vi "Test.vi"   [LabVIEW 2018]
doc: "This VI is called when test mode begins, and will automatically be terminated when it ends. You can add manual or automatic tests and invoke them from the dashboard."
uses:
  <vilib>/Rock Robotics/WPI/ThirdParty/Phoenix-LabVIEW/Motor Controller/Controls/CTRE_Phoenix_MotorControl_ControlMode.ctl
  <vilib>/Rock Robotics/WPI/Utilities/WPI_GetSetVariantRefNum.vi
  <vilib>/Rock Robotics/Network Tables/NT Read Number.vi
  <vilib>/Rock Robotics/WPI/RobotDrive/WPI_RobotDriveArcadeDrive_Standard(NoSaturation).vi
types:
  T1 = typedef "WPI_RobotDriveDevRef.ctl" = cluster{"DevStatus":errorcluster, "Motors[]":T2[], "Square Inputs":bool, "Max Output":dbl}
  T2 = typedef "WPI_MotorControlDeviceRef.ctl" = cluster{"DeviceStatus":errorcluster, "Type":T3, "PWM":cluster{"PWM Channel":T4, "DeadBand":T5}, "CAN":cluster{"Device Number":u8, "SetOutput VI Ref":variant, "GetOutput VI Ref":variant, "Enable VI Ref":variant, "Disable VI Ref":variant, "Data":variant}, "Invert":bool, "DIO PWM":cluster{"PWM \"Enable\" Channel":T4, "DIOChannel":T6, "PWM Rate":dbl}}
  T3 = typedef "WPI_MotorControlType.ctl" = enum16{"PWM", "CAN", "DIO PWM"}
  T4 = typedef "FPGA_DIOPWMChannel.ctl" = enum8{"PWM 0", "PWM 1", "PWM 2", "PWM 3", "PWM 4", "PWM 5", "PWM 6", "PWM 7", "PWM 8", "PWM 9", "PWM MXP 0", "PWM MXP 1", "PWM MXP 2", "PWM MXP 3", "PWM MXP 4", "PWM MXP 5", "PWM MXP 6", "PWM MXP 7", "PWM MXP 8", "PWM MXP 9", "Invalid"}
  T5 = typedef "WPI_PWMDeadband.ctl" = cluster{"Name":string, "maxPositivePwm":i32, "minPositivePwm":i32, "centerPwm":i32, "maxNegativePwm":i32, "minNegativePwm":i32, "angularRange":u16}
  T6 = typedef "FPGA_DIOChannel.ctl" = enum8{"DIO 0", "DIO 1", "DIO 2", "DIO 3", "DIO 4", "DIO 5", "DIO 6", "DIO 7", "DIO 8", "DIO 9", "DIO MXP 0", "DIO MXP 1", "DIO MXP 2", "DIO MXP 3", "DIO MXP 4", "DIO MXP 5", "DIO MXP 6", "DIO MXP 7", "DIO MXP 8", "DIO MXP 9", "DIO MXP 10", "DIO MXP 11", "DIO MXP 12", "DIO MXP 13", "DIO MXP 14", "DIO MXP 15", "SPI Port CS1", "SPI Port CS2", "SPI Port CS3", "SPI Port MISO", "SPI Port MOSI", "Invalid"}
  T7 = typedef "WPI_JoystickDevRef.ctl" = cluster{"Device":T8}
  T8 = typedef "WPI_JoystickDeviceEnum.ctl" = enum16{"USB 0", "USB 1", "USB 2", "USB 3", "USB 4", "USB 5"}
  T9 = cluster{"PhoenixMotorControlDevRef":T2, "PhoenixMotorControlDevRef":T2, "PhoenixMotorControlDevRef":T2, "MotorControlDevRef":T2, "MotorControlDevRef":T2, "RobotDriveDevRef":T1, "JoystickDevRef":T7}
  T10 = typedef "CTRE_Phoenix_MotorControl_ControlMode.ctl" = u16
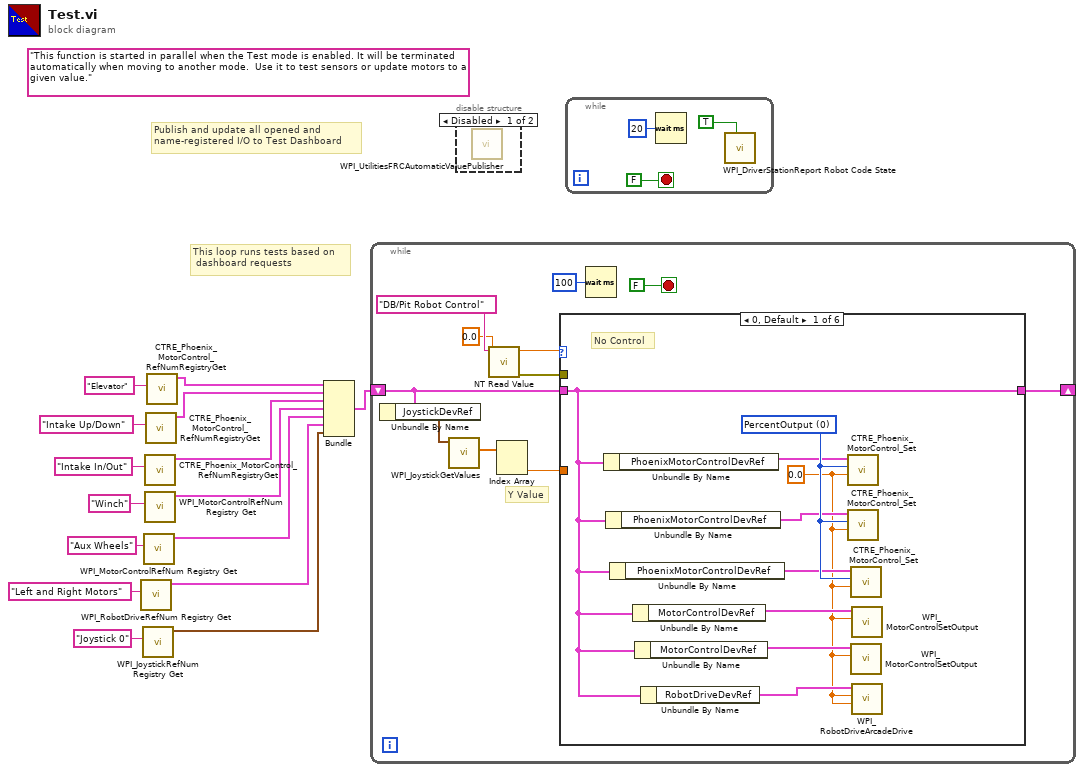
[diagram p0: block diagram]
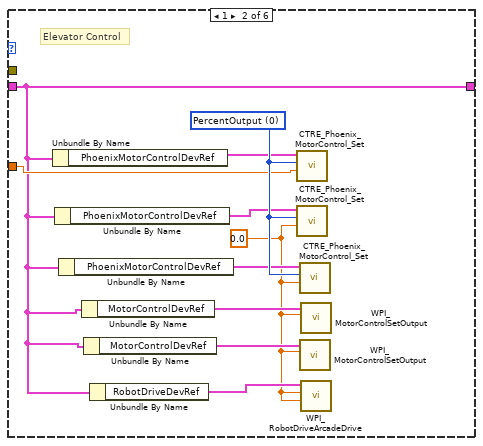
[diagram p2: hidden frame]
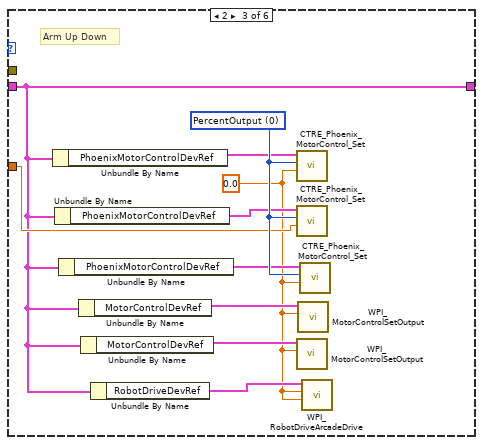
[diagram p3: hidden frame]
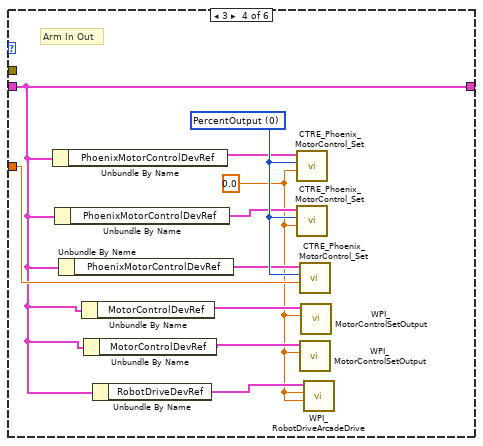
[diagram p4: hidden frame]
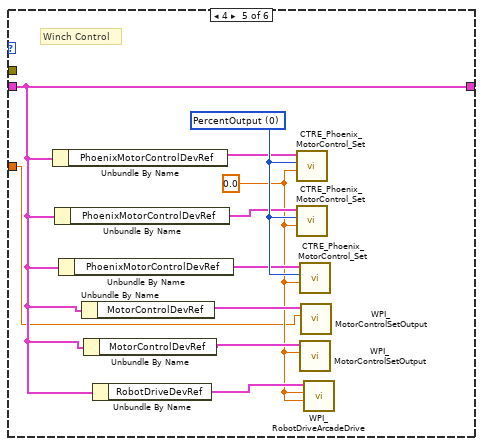
[diagram p5: hidden frame]
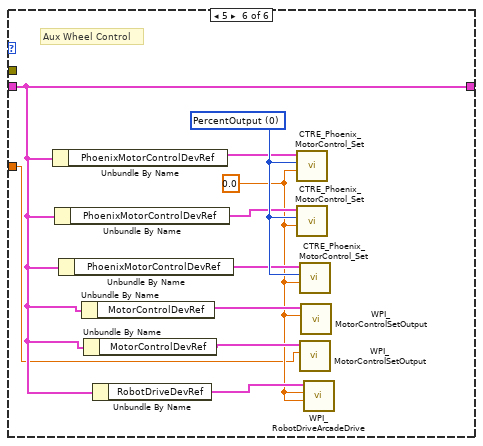
[diagram p6: hidden frame]
diagram:
  (unwired) "This function is started in parallel when the Test mode is enabled. It will be terminated automatically when moving to another mode.  Use it to test sensors or update motors to a given value."
  # "This loop runs tests based on \n dashboard requests"
  # "Publish and update all opened and\nname-registered I/O to Test Dashboard"
  n1 = call <vilib>:"WPI_RobotDriveRefNum Registry Get.vi"("refnum name"="Left and Right Motors") -> ("RobotDriveDevRef"=w6:T1)  [unwired: 9 in, 1 out]
  n2 = call <vilib>:"WPI_JoystickRefNum Registry Get.vi"("refnum name"="Joystick 0") -> ("JoystickDevRef"=w5:T7)  [unwired: 1 in, 9 out]
  n3 = call <vilib>:"WPI_MotorControlRefNum Registry Get.vi"("refnum name"="Aux Wheels") -> ("MotorControlDevRef"=w1:T2)  [unwired: 9 in, 1 out]
  n4 = call <vilib>:"CTRE_Phoenix_MotorControl_RefNumRegistryGet.vi"("refnum name"="Intake In/Out") -> ("PhoenixMotorControlDevRef"=w7:T2)  [unwired: 9 in, 1 out]
  n5 = call <vilib>:"WPI_MotorControlRefNum Registry Get.vi"("refnum name"="Winch") -> ("MotorControlDevRef"=w2:T2)  [unwired: 9 in, 1 out]
  n6 = call <vilib>:"CTRE_Phoenix_MotorControl_RefNumRegistryGet.vi"("refnum name"="Intake Up/Down") -> ("PhoenixMotorControlDevRef"=w8:T2)  [unwired: 9 in, 1 out]
  n7 = call <vilib>:"CTRE_Phoenix_MotorControl_RefNumRegistryGet.vi"("refnum name"="Elevator") -> ("PhoenixMotorControlDevRef"=w12:T2)  [unwired: 9 in, 1 out]
  n8 = Bundle("PhoenixMotorControlDevRef"=w12, "PhoenixMotorControlDevRef"=w8, "PhoenixMotorControlDevRef"=w7, "MotorControlDevRef"=w2, "MotorControlDevRef"=w1, "RobotDriveDevRef"=w6, "JoystickDevRef"=w5) -> (w13:T9)  [unwired: 1 in]
  n9 = while {
    shift-right: [w22] -> _
    shift-left: w13 -> [w19]
    stop <- FALSE stop-if-true
    # "Y Value"
    n10 = Unbundle By Name(w19) -> ("JoystickDevRef"=w18:T7)
    n11 = call <vilib>:"WPI_JoystickGetValues.vi"("JoystickDevRef"=w18) -> ("Axes"=w17:dbl[])  [unwired: 6 in, 4 out]
    n12 = call-poly <vilib>:"NT Read Value.vi"("Default Value"=0.0, "Name"="DB/Pit Robot Control") -> ("error out"=w23:errorcluster, "Numeric"=w24:dbl)  [unwired: 8 in]
    n13 = Index Array(array=w17) -> (element #2=w16:dbl)  [unwired: 2 in, 1 out]
    n14 = case shown="0, Default" w24 {
      tunnel: w23 -> [_ _ _ _ _ _]
      tunnel: w19 -> [w27 w39 w49 w59 w70 w80]
      tunnel: [w27 w39 w49 w59 w70 w80] -> w22
      tunnel: w16 -> [_ w40 w50 w60 w66 w76]
      frame 0, Default {
        w28 = 0.0 ("Output")
        w35 = T10 0 items=["PercentOutput"=0, "Position"=1, "Velocity"=2, "Current"=3, "Follower"=5, "MotionProfile"=6, "MotionMagic"=7, "MotionProfileArc"=10, "Disabled"=15] ("Control Mode")
        # "No Control"
        n15 = Unbundle By Name(w27) -> ("PhoenixMotorControlDevRef"=w34:T2)
        n16 = Unbundle By Name(w27) -> ("PhoenixMotorControlDevRef"=w31:T2)
        n17 = Unbundle By Name(w27) -> ("PhoenixMotorControlDevRef"=w32:T2)
        n18 = Unbundle By Name(w27) -> ("MotorControlDevRef"=w30:T2)
        n19 = Unbundle By Name(w27) -> ("MotorControlDevRef"=w29:T2)
        n20 = Unbundle By Name(w27) -> ("RobotDriveDevRef"=w33:T1)
        n21 = call <vilib>:"CTRE_Phoenix_MotorControl_Set.vi"("Output"=w28, "Control Mode"=w35, "PhoenixMotorControlDevRef"=w34) -> ()  [unwired: 7 in, 2 out]
        n22 = call <vilib>:"CTRE_Phoenix_MotorControl_Set.vi"("Output"=w28, "Control Mode"=w35, "PhoenixMotorControlDevRef"=w31) -> ()  [unwired: 7 in, 2 out]
        n23 = call <vilib>:"CTRE_Phoenix_MotorControl_Set.vi"("Output"=w28, "Control Mode"=w35, "PhoenixMotorControlDevRef"=w32) -> ()  [unwired: 7 in, 2 out]
        n24 = call <vilib>:"WPI_MotorControlSetOutput.vi"("Output"=w28, "MotorControlDevRef"=w29) -> ()  [unwired: 7 in, 3 out]
        n25 = call <vilib>:"WPI_MotorControlSetOutput.vi"("Output"=w28, "MotorControlDevRef"=w30) -> ()  [unwired: 7 in, 3 out]
        n26 = call-poly <vilib>:"WPI_RobotDriveArcadeDrive.vi"("Y axis value"=w28, "X axis value"=w28, "RobotDriveDevRef"=w33) -> ()  [unwired: 6 in, 3 out]
      }
      frame 1 {
        w36 = 0.0 ("Output")
        w45 = T10 0 items=["PercentOutput"=0, "Position"=1, "Velocity"=2, "Current"=3, "Follower"=5, "MotionProfile"=6, "MotionMagic"=7, "MotionProfileArc"=10, "Disabled"=15] ("Control Mode")
        # "Elevator Control"
        n27 = Unbundle By Name(w39) -> ("PhoenixMotorControlDevRef"=w44:T2)
        n28 = Unbundle By Name(w39) -> ("PhoenixMotorControlDevRef"=w41:T2)
        n29 = Unbundle By Name(w39) -> ("PhoenixMotorControlDevRef"=w42:T2)
        n30 = Unbundle By Name(w39) -> ("MotorControlDevRef"=w38:T2)
        n31 = Unbundle By Name(w39) -> ("MotorControlDevRef"=w37:T2)
        n32 = Unbundle By Name(w39) -> ("RobotDriveDevRef"=w43:T1)
        n33 = call <vilib>:"CTRE_Phoenix_MotorControl_Set.vi"("Output"=w40, "Control Mode"=w45, "PhoenixMotorControlDevRef"=w44) -> ()  [unwired: 7 in, 2 out]
        n34 = call <vilib>:"CTRE_Phoenix_MotorControl_Set.vi"("Output"=w36, "Control Mode"=w45, "PhoenixMotorControlDevRef"=w41) -> ()  [unwired: 7 in, 2 out]
        n35 = call <vilib>:"CTRE_Phoenix_MotorControl_Set.vi"("Output"=w36, "Control Mode"=w45, "PhoenixMotorControlDevRef"=w42) -> ()  [unwired: 7 in, 2 out]
        n36 = call <vilib>:"WPI_MotorControlSetOutput.vi"("Output"=w36, "MotorControlDevRef"=w37) -> ()  [unwired: 7 in, 3 out]
        n37 = call <vilib>:"WPI_MotorControlSetOutput.vi"("Output"=w36, "MotorControlDevRef"=w38) -> ()  [unwired: 7 in, 3 out]
        n38 = call-poly <vilib>:"WPI_RobotDriveArcadeDrive.vi"("Y axis value"=w36, "X axis value"=w36, "RobotDriveDevRef"=w43) -> ()  [unwired: 6 in, 3 out]
      }
      frame 2 {
        w46 = 0.0 ("Output")
        w55 = T10 0 items=["PercentOutput"=0, "Position"=1, "Velocity"=2, "Current"=3, "Follower"=5, "MotionProfile"=6, "MotionMagic"=7, "MotionProfileArc"=10, "Disabled"=15] ("Control Mode")
        # "Arm Up Down"
        n39 = Unbundle By Name(w49) -> ("PhoenixMotorControlDevRef"=w54:T2)
        n40 = Unbundle By Name(w49) -> ("PhoenixMotorControlDevRef"=w51:T2)
        n41 = Unbundle By Name(w49) -> ("PhoenixMotorControlDevRef"=w52:T2)
        n42 = Unbundle By Name(w49) -> ("MotorControlDevRef"=w47:T2)
        n43 = Unbundle By Name(w49) -> ("MotorControlDevRef"=w48:T2)
        n44 = Unbundle By Name(w49) -> ("RobotDriveDevRef"=w53:T1)
        n45 = call <vilib>:"CTRE_Phoenix_MotorControl_Set.vi"("Output"=w46, "Control Mode"=w55, "PhoenixMotorControlDevRef"=w54) -> ()  [unwired: 7 in, 2 out]
        n46 = call <vilib>:"CTRE_Phoenix_MotorControl_Set.vi"("Output"=w50, "Control Mode"=w55, "PhoenixMotorControlDevRef"=w51) -> ()  [unwired: 7 in, 2 out]
        n47 = call <vilib>:"WPI_MotorControlSetOutput.vi"("Output"=w46, "MotorControlDevRef"=w48) -> ()  [unwired: 7 in, 3 out]
        n48 = call <vilib>:"WPI_MotorControlSetOutput.vi"("Output"=w46, "MotorControlDevRef"=w47) -> ()  [unwired: 7 in, 3 out]
        n49 = call <vilib>:"CTRE_Phoenix_MotorControl_Set.vi"("Output"=w46, "Control Mode"=w55, "PhoenixMotorControlDevRef"=w52) -> ()  [unwired: 7 in, 2 out]
        n50 = call-poly <vilib>:"WPI_RobotDriveArcadeDrive.vi"("Y axis value"=w46, "X axis value"=w46, "RobotDriveDevRef"=w53) -> ()  [unwired: 6 in, 3 out]
      }
      frame 3 {
        w56 = 0.0 ("Output")
        w65 = T10 0 items=["PercentOutput"=0, "Position"=1, "Velocity"=2, "Current"=3, "Follower"=5, "MotionProfile"=6, "MotionMagic"=7, "MotionProfileArc"=10, "Disabled"=15] ("Control Mode")
        # "Arm In Out"
        n51 = Unbundle By Name(w59) -> ("PhoenixMotorControlDevRef"=w64:T2)
        n52 = Unbundle By Name(w59) -> ("PhoenixMotorControlDevRef"=w61:T2)
        n53 = Unbundle By Name(w59) -> ("PhoenixMotorControlDevRef"=w62:T2)
        n54 = Unbundle By Name(w59) -> ("MotorControlDevRef"=w57:T2)
        n55 = Unbundle By Name(w59) -> ("MotorControlDevRef"=w58:T2)
        n56 = Unbundle By Name(w59) -> ("RobotDriveDevRef"=w63:T1)
        n57 = call <vilib>:"CTRE_Phoenix_MotorControl_Set.vi"("Output"=w56, "Control Mode"=w65, "PhoenixMotorControlDevRef"=w64) -> ()  [unwired: 7 in, 2 out]
        n58 = call <vilib>:"CTRE_Phoenix_MotorControl_Set.vi"("Output"=w56, "Control Mode"=w65, "PhoenixMotorControlDevRef"=w61) -> ()  [unwired: 7 in, 2 out]
        n59 = call <vilib>:"CTRE_Phoenix_MotorControl_Set.vi"("Output"=w60, "Control Mode"=w65, "PhoenixMotorControlDevRef"=w62) -> ()  [unwired: 7 in, 2 out]
        n60 = call <vilib>:"WPI_MotorControlSetOutput.vi"("Output"=w56, "MotorControlDevRef"=w58) -> ()  [unwired: 7 in, 3 out]
        n61 = call <vilib>:"WPI_MotorControlSetOutput.vi"("Output"=w56, "MotorControlDevRef"=w57) -> ()  [unwired: 7 in, 3 out]
        n62 = call-poly <vilib>:"WPI_RobotDriveArcadeDrive.vi"("Y axis value"=w56, "X axis value"=w56, "RobotDriveDevRef"=w63) -> ()  [unwired: 6 in, 3 out]
      }
      frame 4 {
        w67 = 0.0 ("Output")
        w75 = T10 0 items=["PercentOutput"=0, "Position"=1, "Velocity"=2, "Current"=3, "Follower"=5, "MotionProfile"=6, "MotionMagic"=7, "MotionProfileArc"=10, "Disabled"=15] ("Control Mode")
        # "Winch Control"
        n63 = Unbundle By Name(w70) -> ("PhoenixMotorControlDevRef"=w74:T2)
        n64 = Unbundle By Name(w70) -> ("PhoenixMotorControlDevRef"=w71:T2)
        n65 = Unbundle By Name(w70) -> ("PhoenixMotorControlDevRef"=w72:T2)
        n66 = Unbundle By Name(w70) -> ("MotorControlDevRef"=w68:T2)
        n67 = Unbundle By Name(w70) -> ("MotorControlDevRef"=w69:T2)
        n68 = Unbundle By Name(w70) -> ("RobotDriveDevRef"=w73:T1)
        n69 = call <vilib>:"CTRE_Phoenix_MotorControl_Set.vi"("Output"=w67, "Control Mode"=w75, "PhoenixMotorControlDevRef"=w74) -> ()  [unwired: 7 in, 2 out]
        n70 = call <vilib>:"CTRE_Phoenix_MotorControl_Set.vi"("Output"=w67, "Control Mode"=w75, "PhoenixMotorControlDevRef"=w71) -> ()  [unwired: 7 in, 2 out]
        n71 = call <vilib>:"CTRE_Phoenix_MotorControl_Set.vi"("Output"=w67, "Control Mode"=w75, "PhoenixMotorControlDevRef"=w72) -> ()  [unwired: 7 in, 2 out]
        n72 = call <vilib>:"WPI_MotorControlSetOutput.vi"("Output"=w67, "MotorControlDevRef"=w69) -> ()  [unwired: 7 in, 3 out]
        n73 = call <vilib>:"WPI_MotorControlSetOutput.vi"("Output"=w66, "MotorControlDevRef"=w68) -> ()  [unwired: 7 in, 3 out]
        n74 = call-poly <vilib>:"WPI_RobotDriveArcadeDrive.vi"("Y axis value"=w67, "X axis value"=w67, "RobotDriveDevRef"=w73) -> ()  [unwired: 6 in, 3 out]
      }
      frame 5 {
        w77 = 0.0 ("Output")
        w85 = T10 0 items=["PercentOutput"=0, "Position"=1, "Velocity"=2, "Current"=3, "Follower"=5, "MotionProfile"=6, "MotionMagic"=7, "MotionProfileArc"=10, "Disabled"=15] ("Control Mode")
        # "Aux Wheel Control"
        n75 = Unbundle By Name(w80) -> ("PhoenixMotorControlDevRef"=w84:T2)
        n76 = Unbundle By Name(w80) -> ("PhoenixMotorControlDevRef"=w81:T2)
        n77 = Unbundle By Name(w80) -> ("PhoenixMotorControlDevRef"=w82:T2)
        n78 = Unbundle By Name(w80) -> ("MotorControlDevRef"=w78:T2)
        n79 = Unbundle By Name(w80) -> ("MotorControlDevRef"=w79:T2)
        n80 = Unbundle By Name(w80) -> ("RobotDriveDevRef"=w83:T1)
        n81 = call <vilib>:"CTRE_Phoenix_MotorControl_Set.vi"("Output"=w77, "Control Mode"=w85, "PhoenixMotorControlDevRef"=w84) -> ()  [unwired: 7 in, 2 out]
        n82 = call <vilib>:"CTRE_Phoenix_MotorControl_Set.vi"("Output"=w77, "Control Mode"=w85, "PhoenixMotorControlDevRef"=w81) -> ()  [unwired: 7 in, 2 out]
        n83 = call <vilib>:"CTRE_Phoenix_MotorControl_Set.vi"("Output"=w77, "Control Mode"=w85, "PhoenixMotorControlDevRef"=w82) -> ()  [unwired: 7 in, 2 out]
        n84 = call <vilib>:"WPI_MotorControlSetOutput.vi"("Output"=w76, "MotorControlDevRef"=w79) -> ()  [unwired: 7 in, 3 out]
        n85 = call <vilib>:"WPI_MotorControlSetOutput.vi"("Output"=w77, "MotorControlDevRef"=w78) -> ()  [unwired: 7 in, 3 out]
        n86 = call-poly <vilib>:"WPI_RobotDriveArcadeDrive.vi"("Y axis value"=w77, "X axis value"=w77, "RobotDriveDevRef"=w83) -> ()  [unwired: 6 in, 3 out]
      }
    }
    n87 = Wait (ms)(milliseconds to wait=u32 100) -> ()  [unwired: 1 out]
  }
  n88 = disable-structure shown="Disabled" {
    frame Disabled {
      n89 = call <vilib>:"WPI_UtilitiesFRCAutomaticValuePublisher.vi"() -> ()  [unwired: 12 in]
    }
    frame Enabled {
    }
  }
  n90 = while {
    stop <- FALSE stop-if-true
    n91 = Wait (ms)(milliseconds to wait=u32 20) -> ()  [unwired: 1 out]
    n92 = call <vilib>:"WPI_DriverStationReport Robot Code State.vi"("Test"=TRUE ("Autonomous")) -> ()  [unwired: 10 in, 1 out]
  }
